vi "test Value in Range (U16).vi"(8 "error in":errorcluster, 11 "TestCase in":refnum<class "SharedUtilities.lvclass">=refnum) -> (0 "error out":errorcluster, 3 "TestCase out":refnum<class "SharedUtilities.lvclass">)   [LabVIEW 2021, in "SharedUtilities.lvclass"]
uses:
  SharedUtilities.lvclass
  d420cf22-d88b-4d62-b1d6-379cc04e7321.vi
  52802dbc-dbe3-43c0-91ad-fe6bb3ee3cf0.vi
  2354b3b9-385b-4659-8e68-155b7c3ecaba.vi
  5cac29be-b20d-407d-8ce7-3adecf71f1cb.vi
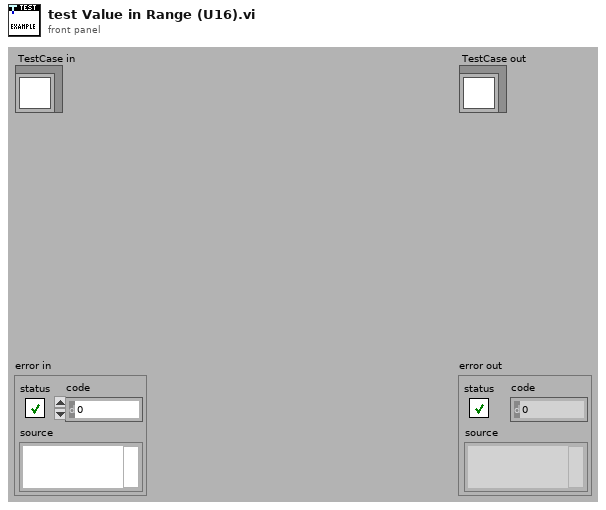
[diagram p1: front panel]
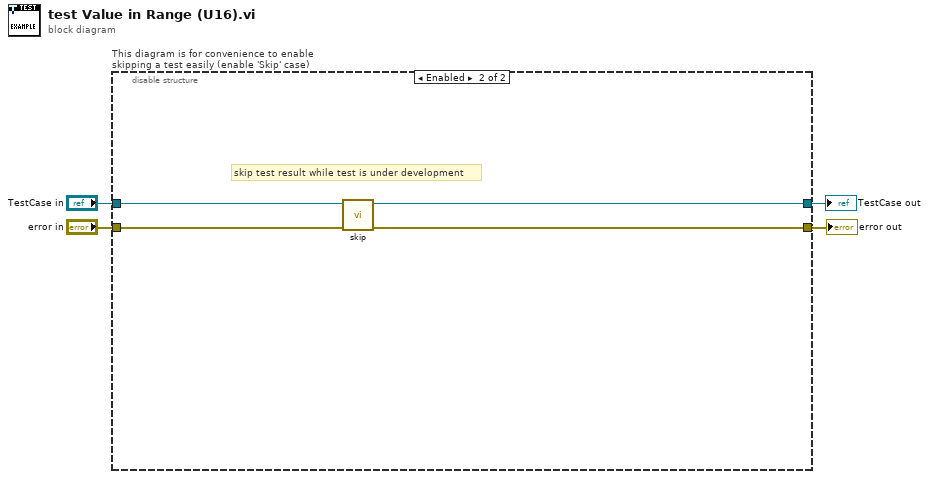
[diagram p0: block diagram]
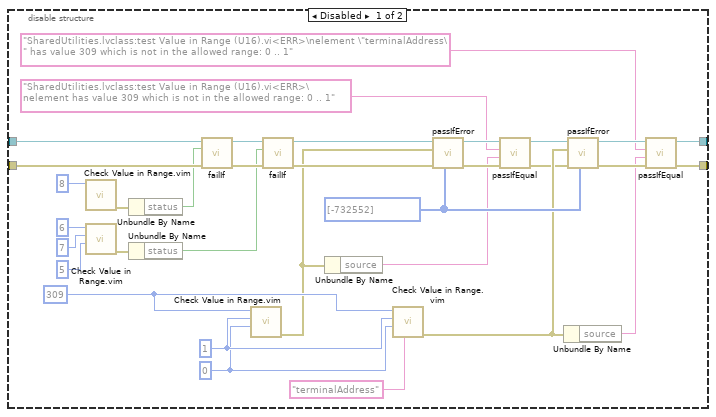
[diagram p2: hidden frame]
diagram:
  n1 = disable-structure "This diagram is for convenience to enable skipping a test easily (enable 'Skip' case)" shown="Enabled" {
    disable-tunnel: "TestCase in" -> [w33 w41]
    disable-tunnel: [w10 w39] -> w1
    disable-tunnel: [w11 w40] -> w3
    disable-tunnel: "error in" -> [w32 w38]
    frame Disabled {
      w20 = i32[] [-732552] ("passing error codes (default = any error code)")
      w27 = i8 0
      w28 = u8 1
      w21 = u16 309
      n2 = call "Check Value in Range.vim"("value"=u16 8) -> ("error out"=w25:errorcluster)  [unwired: 10 in]
      n3 = call "Check Value in Range.vim"("lower limit (0)"=u16 5, "upper limit (31)"=u16 7, "value"=u16 6) -> ("error out"=w23:errorcluster)  [unwired: 8 in]
      n4 = Unbundle By Name(w25) -> ("status"=w24:bool)
      n5 = Unbundle By Name(w23) -> ("status"=w22:bool)
      n6 = call-dynamic "failIf.vi"("error in (no error)"=w32, "fail"=w24, "TestCase in"=w33) -> ("error out"=w35:errorcluster, "TestCase out"=w34:refnum<class "SharedUtilities.lvclass">)  [unwired: 7 in]
      n7 = call "Check Value in Range.vim"("lower limit (0)"=w27, "upper limit (31)"=w28, "value"=w21) -> ("error out"=w18:errorcluster)  [unwired: 8 in]
      n8 = call-dynamic "failIf.vi"("error in (no error)"=w35, "fail"=w22, "TestCase in"=w34) -> ("error out"=w37:errorcluster, "TestCase out"=w36:refnum<class "SharedUtilities.lvclass">)  [unwired: 7 in]
      n9 = Unbundle By Name(w18) -> ("source"=w9:string)
      n10 = call "Check Value in Range.vim"("element name"="terminalAddress", "lower limit (0)"=w27, "upper limit (31)"=w28, "value"=w21) -> ("error out"=w19:errorcluster)  [unwired: 7 in]
      n11 = call-dynamic "passIfError.vi"("passing error codes (default = any error code)"=w20, "error in (no error)"=w37, "error"=w18, "TestCase in"=w36) -> ("error out"=w17:errorcluster, "TestCase out"=w16:refnum<class "SharedUtilities.lvclass">)  [unwired: 6 in]
      n12 = call-dynamic "passIfEqual.vi"("error in (no error)"=w17, "y"=w9, "x"="SharedUtilities.lvclass:test Value in Range (U16).vi<ERR>\nelement has value 309 which is not in the allowed range: 0 .. 1" ("Display"), "TestCase in"=w16) -> ("error out"=w14:errorcluster, "TestCase out"=w15:refnum<class "SharedUtilities.lvclass">)  [unwired: 6 in]
      n13 = Unbundle By Name(w19) -> ("source"=w8:string)
      n14 = call-dynamic "passIfError.vi"("passing error codes (default = any error code)"=w20, "error in (no error)"=w14, "error"=w19, "TestCase in"=w15) -> ("error out"=w12:errorcluster, "TestCase out"=w13:refnum<class "SharedUtilities.lvclass">)  [unwired: 6 in]
      n15 = call-dynamic "passIfEqual.vi"("error in (no error)"=w12, "y"=w8, "x"="SharedUtilities.lvclass:test Value in Range (U16).vi<ERR>\nelement \"terminalAddress\" has value 309 which is not in the allowed range: 0 .. 1" ("Display"), "TestCase in"=w13) -> ("error out"=w11:errorcluster, "TestCase out"=w10:refnum<class "SharedUtilities.lvclass">)  [unwired: 6 in]
    }
    frame Enabled {
      # "skip test result while test is under development"
      n16 = call <vilib>:"skip.vi"("error in (no error)"=w38, "TestCase in"=w41) -> ("error out"=w40:errorcluster, "TestCase out"=w39:refnum<class "SharedUtilities.lvclass">)  [unwired: 8 in]
    }
  }
  "error out" <- w3
  "TestCase out" <- w1
